vi "FilterGlyphs.vi"(8 "error in (no error)":errorcluster, 9 "DNL_Glyphs []":refnum<vi>, 10 "Tag":string, 11 "Glyph in":refnum<class "Glyph.lvclass">) -> (0 "error out":errorcluster, 3 "Glyph out":refnum<class "Glyph.lvclass">)   [LabVIEW 2021, in "Glyph.lvclass"]
uses:
  <resource>/plugins/NIIconEditor/Class/Icon Library/Glyph.lvclass
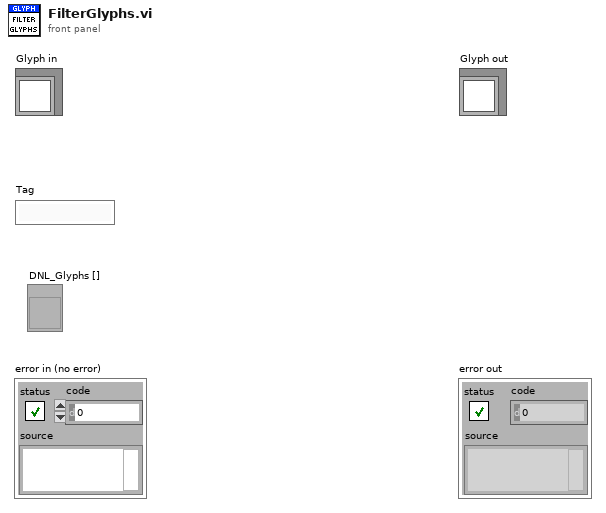
[diagram p1: front panel]
types:
  T1 = typedef "Graphic.ctl" = cluster{"Rectangle":cluster{"left":i16, "top":i16, "right":i16, "bottom":i16}, "Path":path, "Image":picture, "Filter":string, "FileName":string}
  T2 = typedef "Path&Icon.ctl" = cluster{"Rectangle":cluster{"left":i16, "top":i16, "right":i16, "bottom":i16}, "Path":path, "Image":picture, "Filter":string, "FileName":string}
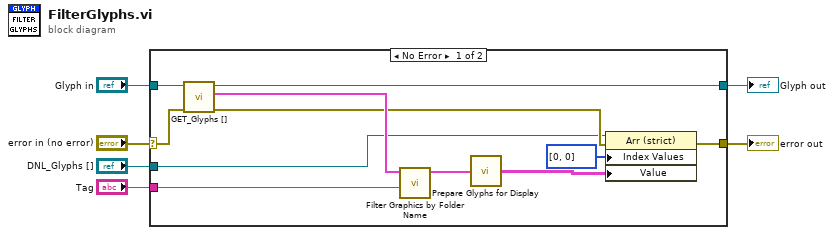
[diagram p0: block diagram]
diagram:
  n1 = case shown="No Error" "error in (no error)" {
    selector: "error in (no error)" -> [w14 w19]
    tunnel: [w17 w19] -> w5
    tunnel: [w15 w18] -> w3
    tunnel: "Glyph in" -> [w16 w18]
    tunnel: "Tag" -> [w7 _]
    tunnel: "DNL_Glyphs []" -> [w8 _]
    frame No Error {
      n2 = call-dynamic "GET_Glyphs [].vi"("error in (no error)"=w14, "Glyph.lvclass in"=w16) -> ("error out"=w9:errorcluster, "Glyphs []"=w13:T1[], "Glyph.lvclass out"=w15:refnum<class "Glyph.lvclass">)  [unwired: 7 out]
      n3 = call <resource>:"Filter Graphics by Folder Name.vi"("Tag"=w7, "Glyphs [] in"=w13) -> ("Filtered Glyphs []"=w12:T1[])  [unwired: 9 out]
      n4 = call <resource>:"Prepare Glyphs for Display.vi"("Icon Templates"=w12) -> ("Array"=w10:T2[][])
      n5 = property class="Arr (strict)"(reference=w8, error in=w9, "Index Values"=u32[] [0, 0], "Value"=w10) -> (error out=w17:errorcluster)  [unwired: 1 out]
    }
    frame Error {
    }
  }
  "error out" <- w5
  "Glyph out" <- w3
